vi "TSE Deneme.vi"() -> ()   [LabVIEW 2014]
uses:
  CustomControls/TSE_Status.ctl
  CustomControls/Program_States.ctl
panel:
  out "Uygulanan_Deger":dbl[](array[numeric])
  out "TSE Status":T1={"Return Code"=0, "Message"="", "error in (no error)"={"status"=FALSE, "code"=0, "source"=""}, "Program State"=enum."Ön Yükleme Tamam", "Test A. Suresi"=0}
  in  "StopTSE":bool
  in  "ExecuteTest":bool
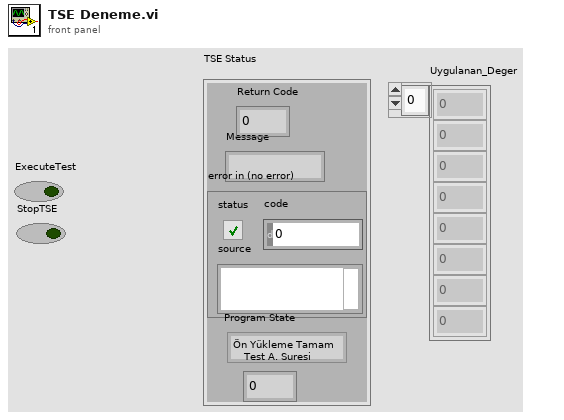
[diagram p1: front panel]
types:
  T1 = typedef "TSE_Status.ctl" = cluster{"Return Code":i32, "Message":string, "error in (no error)":errorcluster, "Program State":T2, "Test A. Suresi":u32}
  T2 = typedef "Program_States.ctl" = enum16{"Ön Yükleme", "TSE Baslat", "Kalibratöre Baglan", "Kalibratörü Baslat", "Ön Yükleme Tamam", "Frekans Testi", "Gerilim Testi", "Akim Testi", "Aktif Guc Testi", "Reaktif Guc Testi", "AC Akim Harmonik Testi", "AC Gerilim Harmonik Testi", "Flicker Testi", "Rapor Cikarma", "Yeniden Başlat", "Bekleme", "Durdur"}
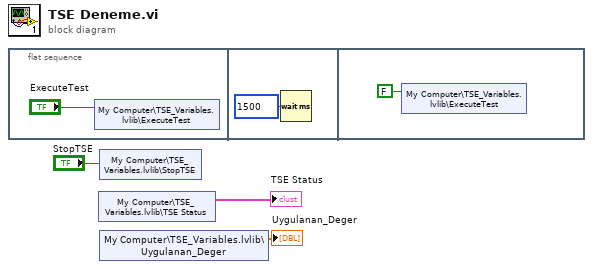
[diagram p0: block diagram]
diagram:
  n1 = flat-sequence {
    frame #0 {
      n2 = shared-variable "My Computer\\TSE_Variables.lvlib\\ExecuteTest"("ExecuteTest") -> ()  [unwired: 1 in, 1 out]
    }
    frame #1 {
      n3 = Wait (ms)(milliseconds to wait=u32 1500) -> ()  [unwired: 1 out]
    }
    frame #2 {
      n4 = shared-variable "My Computer\\TSE_Variables.lvlib\\ExecuteTest"(FALSE ("ExecuteTest")) -> ()  [unwired: 1 in, 1 out]
    }
  }
  n5 = shared-variable "My Computer\\TSE_Variables.lvlib\\TSE Status"() -> (→"TSE Status":T1)  [unwired: 1 in, 1 out]
  n6 = shared-variable "My Computer\\TSE_Variables.lvlib\\StopTSE"("StopTSE") -> ()  [unwired: 1 in, 1 out]
  n7 = shared-variable "My Computer\\TSE_Variables.lvlib\\Uygulanan_Deger"() -> (→"Uygulanan_Deger":dbl[])  [unwired: 1 in, 1 out]
